vi "Test DAQ.vi"() -> ()   [LabVIEW 2019, in "Instrument.Lockin.lvlib" / "Instrument.DAQ.lvclass"]
uses:
  Instrument.DAQ.lvclass
  Typedefs/AO.Channel--Cluster--Array.ctl
  Typedefs/AO.Channel--Cluster.ctl
  Typedefs/AO.Channel.Function--Enum.ctl
  Typedefs/DAQ.Config.AI--Cluster.ctl
  Typedefs/DAQ.Config.AI.Coupling--enum.ctl
  Typedefs/DAQ.Config.AI.Range--enum.ctl
  Typedefs/DAQ.Type--enum.ctl
  Typedefs/DAQ.Config.AO--Cluster.ctl
  Typedefs/DAQ.Config.AO.Range--enum.ctl
  Typedefs/DAQ.Sampling.Sampling--Cluster.ctl
  Instrument.DAQ.lvclass/Instrument.DAQ.ctl
panel:
  out "error out":errorcluster
  in  "Configuration.Channels.Cfg_AO":T1 {"Phase" format="%#_3g"; "Frequency" min=0.0001 max=200000.0 format="%#_6p"; "Offset" format="%#_6p"; "Amplitude" min=0.0 max=10.0 format="%#_6p"}
  out "Waveform Graph":dbl[][](graph)
  in  "stop":bool
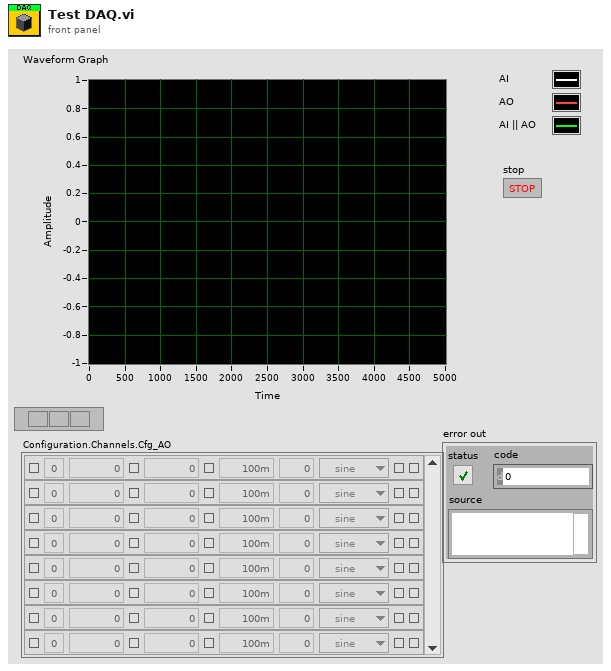
[diagram p1: front panel]
types:
  T1 = typedef "Instrument.Lockin.lvlib/Instrument.DAQ.lvclass/AO.Channel--Cluster--Array.ctl" = T2[]
  T2 = typedef "Instrument.Lockin.lvlib/Instrument.DAQ.lvclass/AO.Channel--Cluster.ctl" = cluster{"Enable?":bool, "Channel":i32, "Amplitude":dbl, "Offset":dbl, "Frequency":dbl, "Phase":dbl, "Function":T3, "Sweeping?":bool, "Limit AC":bool, "Limit DC?":bool, "Duty Cycle":bool}
  T3 = typedef "Instrument.Lockin.lvlib/Instrument.DAQ.lvclass/AO.Channel.Function--Enum.ctl" = enum16{"sine", "square", "triangle", "saw"}
  T4 = typedef "Instrument.Lockin.lvlib/Instrument.DAQ.lvclass/DAQ.Sampling.Sampling--Cluster.ctl" = cluster{"Fs":dbl, "#s":i32}
  T5 = typedef "Instrument.Lockin.lvlib/Instrument.DAQ.lvclass/DAQ.Config.AO--Cluster.ctl" = cluster{"Channels":tag, "Range":T6, "output terminal configuration":i32, "Type":T7}
  T6 = typedef "Instrument.Lockin.lvlib/Instrument.DAQ.lvclass/DAQ.Config.AO.Range--enum.ctl" = enum16{"±0.1", "±1.0", "±3.5", "±10.0", ""}
  T7 = typedef "Instrument.Lockin.lvlib/Instrument.DAQ.lvclass/DAQ.Type--enum.ctl" = enum16{"None", "USB-4431", "PXI-446x"}
  T8 = typedef "Instrument.Lockin.lvlib/Instrument.DAQ.lvclass/DAQ.Config.AI--Cluster.ctl" = cluster{"Channels":tag, "Coupling":T9, "Range":T10, "input terminal configuration":i32, "Type":T7}
  T9 = typedef "Instrument.Lockin.lvlib/Instrument.DAQ.lvclass/DAQ.Config.AI.Coupling--enum.ctl" = u16
  T10 = typedef "Instrument.Lockin.lvlib/Instrument.DAQ.lvclass/DAQ.Config.AI.Range--enum.ctl" = enum16{"±0.316", "±1.00", "±3.16", "±10.0", "±31.6", "±42.4", ""}
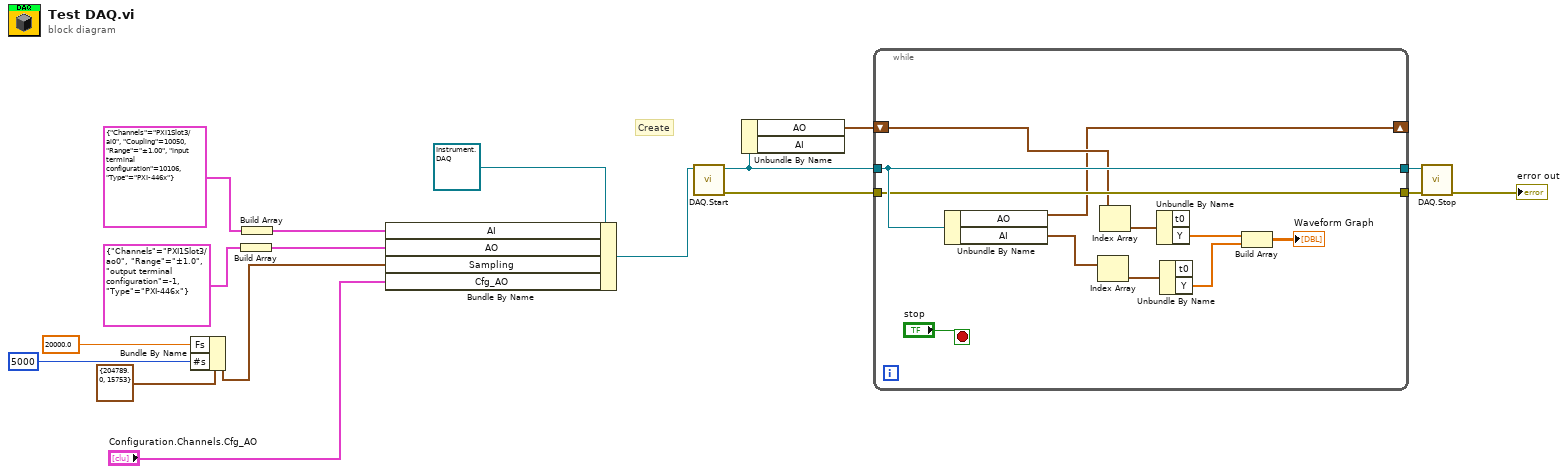
[diagram p0: block diagram]
diagram:
  # "Create"
  n1 = Bundle By Name(cluster=T4 {"Fs"=204789.0, "#s"=15753} ("Configuration.DAQ.Sampling.Sampling"), "Fs"=20000.0, "#s"=5000) -> (w8:T4)
  n2 = Build Array(T5 {"Channels"="PXI1Slot3/ao0", "Range"=enum."±1.0", "output terminal configuration"=-1, "Type"=enum."PXI-446x"} ("AO.config")) -> (w13:T5[])
  n3 = Build Array(T8 {"Channels"="PXI1Slot3/ai0", "Coupling"=10050, "Range"=enum."±1.00", "input terminal configuration"=10106, "Type"=enum."PXI-446x"} ("AI.Config")) -> (w14:T8[])
  n4 = Bundle By Name(cluster=refnum<class "Instrument.DAQ.lvclass"> refnum ("Instrument.DAQ"), "AI"=w14, "AO"=w13, "Sampling"=w8, "Cfg_AO"="Configuration.Channels.Cfg_AO") -> (w16:refnum<class "Instrument.DAQ.lvclass">)
  n5 = call "DAQ.Start.vi"("Instrument.DAQ"=w16) -> ("error out"=w6:errorcluster, "Instrument.DAQ out"=w5:refnum<class "Instrument.DAQ.lvclass">)  [unwired: 9 in]
  n6 = Unbundle By Name(w5) -> ("AO"=w2:waveform(dbl)[])  [unwired: 1 out]
  n7 = while {
    tunnel: w5 -> [w21]
    tunnel: w6 -> [w20]
    shift-right: [w18] -> _
    shift-left: w2 -> [w19]
    tunnel: [w21] -> w3
    tunnel: [w20] -> w4
    stop <- "stop" stop-if-true
    n8 = Unbundle By Name(w21) -> ("AO"=w18:waveform(dbl)[], "AI"=w22:waveform(dbl)[])
    n9 = Index Array(array=w22) -> (element=w26:waveform(dbl))  [unwired: 1 in]
    n10 = Index Array(array=w19) -> (element=w25:waveform(dbl))  [unwired: 1 in]
    n11 = Unbundle By Name(w25) -> ("Y"=w24:dbl[])  [unwired: 1 out]
    n12 = Unbundle By Name(w26) -> ("Y"=w23:dbl[])  [unwired: 1 out]
    n13 = Build Array(w24, w23) -> (→"Waveform Graph":dbl[][])
  }
  n14 = call "DAQ.Stop.vi"("error in (no error)"=w4, "Instrument.DAQ in"=w3) -> ("error out"=→"error out":errorcluster)  [unwired: 8 in, 1 out]
